vi "SubVI Tester.vi"() -> ()   [LabVIEW 2015]
panel:
  out "Warning Text":string="No Warning"
  out "Warning?":bool
  out "Thermometer":dbl(slide) scale=0.0..100.0
  in  "Min Temperature":dbl=10.0
  in  "Max Temperature":dbl=30.0
  in  "Stop":bool
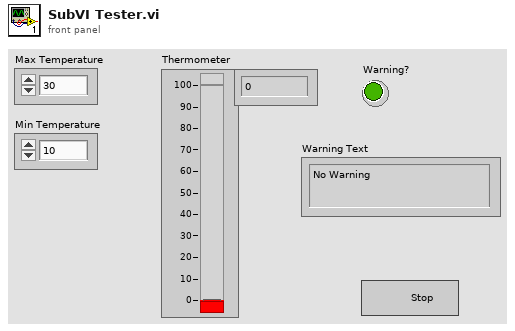
[diagram p1: front panel]
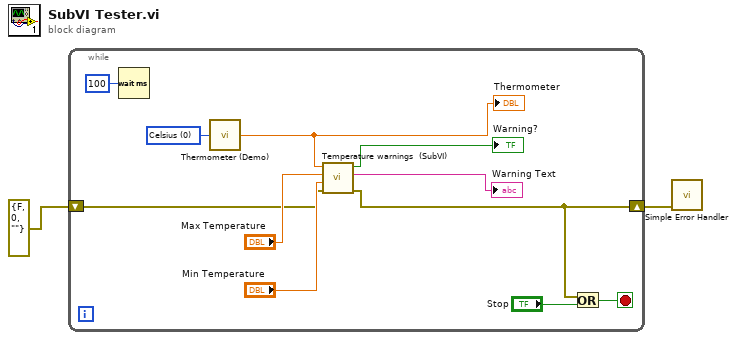
[diagram p0: block diagram]
diagram:
  n1 = while {
    shift-right: [w4] -> w2
    shift-left: errorcluster {"status"=FALSE, "code"=0, "source"=""} ("error in") -> [w7]
    stop <- w11 stop-if-true
    w3 = u16 0 items=["Celsius", "Fahrenheit"] ("Units (0: Celsius)")
    n2 = Wait (ms)(milliseconds to wait=u32 100) -> ()  [unwired: 1 out]
    n3 = call "Thermometer (Demo).vi"("Units (0: Celsius)"=w3) -> ("Temperature Value"=w10:dbl)
    "Thermometer" <- w10
    n4 = call "Temperature warnings  (SubVI).vi"("error in (no error)"=w7, "Min Temperature"="Min Temperature", "Max Temperature"="Max Temperature", "Current Temperature"=w10) -> ("error out"=w4:errorcluster, "f"=→"Warning Text":string, "Boolean"=→"Warning?":bool)  [unwired: 5 in]
    n5 = Or(x=w4, y="Stop") -> (x .or. y?=w11:bool)
  }
  n6 = call <vilib>:"Simple Error Handler.vi"("error in (no error)"=w2) -> ()  [unwired: 4 in, 5 out]
